vi "Return to Thread Pool.vi"(8 "error in (no error)":errorcluster, 11 "Transceiver Thread in":refnum<class "Transceiver Thread.lvclass">) -> (0 "error out":errorcluster, 3 "Transceiver Thread out":refnum<class "Transceiver Thread.lvclass">)   [LabVIEW 2017, in "Data Sharing Framework Core.lvlib" / "Data Sharing Framework Engine.lvlib" / "Transceiver Thread.lvclass"]
uses:
  Transceiver Thread.lvclass
  Transceiver Thread.lvclass/Transceiver Thread.ctl
  Execution/Thread Parameters/Thread Parameters.lvclass/Thread Parameters.ctl
  Execution/Pool/Pool/Pool.lvclass/Pool.ctl
  Debug/Debug Flags FIFO/Debug Flags FIFO.lvclass/Debug Flags FIFO.ctl
  Execution/Pool/Pool/Write FIFO.vi
  Execution/Pool/Pool/Get FIFO.vi
  Execution/Pool/Pool/Get Debug Flags.vi
  Debug/Debug Flags FIFO/Get Infinite Timeouts.vi
  Execution/Pool/Pool ID/Pool ID.lvclass
  C:/github/data-sharing-framework/Source/Data Sharing Framework Core/Engine/Internal/Execution/Pool/Pool/Pool.lvclass
  Execution/Thread Parameters/Thread Parameters.lvclass
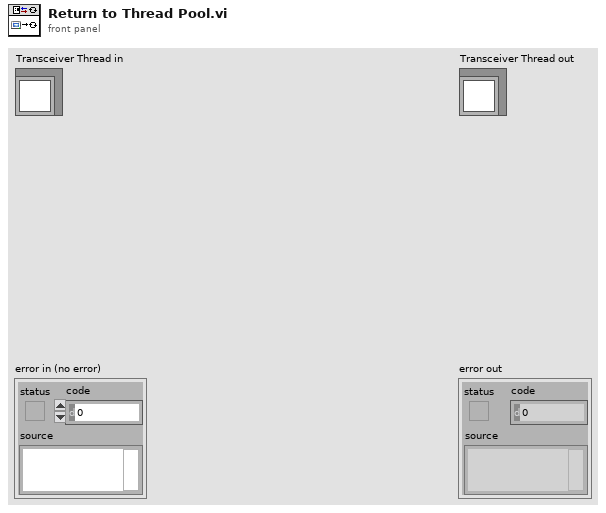
[diagram p1: front panel]
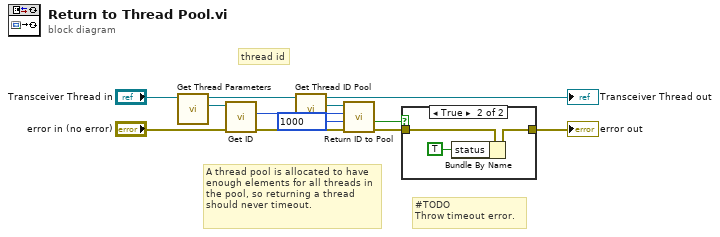
[diagram p0: block diagram]
diagram:
  # "thread id"
  # "A thread pool is allocated to have enough elements for all threads in the pool, so returning a thread should never timeout."
  # "#TODO\nThrow timeout error."
  n1 = call "Get Thread Parameters.vi"("Transceiver Thread in"="Transceiver Thread in") -> ("Thread Parameters"=w4:refnum<class "Thread Parameters.lvclass">, "Transceiver Thread out"=w1:refnum<class "Transceiver Thread.lvclass">)  [unwired: 9 in]
  n2 = call "Get ID.vi"("Plugin in"=w4) -> ("id"=w3:i32)  [unwired: 9 in, 1 out]
  n3 = call "Get Thread ID Pool.vi"("Transceiver Thread in"=w1) -> ("Thread ID Pool"=w11:refnum<class "Pool ID.lvclass">, "Transceiver Thread out"=→"Transceiver Thread out":refnum<class "Transceiver Thread.lvclass">)  [unwired: 9 in]
  n4 = call "Return ID to Pool.vi"("error in (no error)"="error in (no error)", "timeout in ms (0)"=1000, "id"=w3, "ID Pool in"=w11) -> ("error out"=w7:errorcluster, "timed out?"=w6:bool)  [unwired: 5 in, 1 out]
  n5 = case shown="True" w6 {
    tunnel: w7 -> [w12 w15]
    tunnel: [w12 w13] -> w5
    frame False {
    }
    frame True {
      n6 = Bundle By Name(cluster=w15, "status"=TRUE) -> (w13:errorcluster)
    }
  }
  "error out" <- w5
